vi "Actor Core.vi"(8 "error in":errorcluster, 11 "Create Test Channel View in":refnum<class "Create Test Channel View.lvclass">) -> (0 "error out":errorcluster, 3 "Actor out":refnum<class "Actor.lvclass">)   [LabVIEW 2013, in "Create Test Channel View.lvlib" / "Create Test Channel View.lvclass"]
doc: "(<B>Filename</B>: Actor Framework.lvlib:Actor.lvclass:Actor Core.vi)\n\nReceives messages to the actor, reacts to them, and initiates any error handling that may shut the actor down.\n\nDescendant classes may override this VI to append parallel tasks for the actor to complete while it handles messages. Overrides use the Call Parent Method node."
uses:
  Create Test Channel View.lvclass
  <vilib>/ActorFramework/Actor/Actor.lvclass
  <vilib>/ActorFramework/Actor/Actor.lvclass/Actor.ctl
  <vilib>/ActorFrameworkMVC/View Actor/View Actor.lvclass
  <vilib>/ActorFramework/Message Enqueuer/Message Enqueuer.lvclass/Message Enqueuer.ctl
  Create Test Channel View.lvclass/Create Test Channel View.ctl
  <vilib>/Utility/miscctls.llb/LVPositionTypeDef.ctl
  <vilib>/ActorFrameworkMVC/UI Controller Messages/Move Subpanel Msg/Move Subpanel Msg.lvclass/Move Subpanel Msg.ctl
  <vilib>/ActorFrameworkMVC/UI Controller Messages/Insert Subpanel Msg/Insert Subpanel Msg.lvclass/Insert Subpanel Msg.ctl
  Models/Create Test Channel Model Messages/Set Item Configurations Msg/Set Item Configurations Msg.lvclass/Set Item Configurations Msg.ctl
  <vilib>/ActorFramework/Message Enqueuer/Init from Existing Queue.vi
  <vilib>/ActorFramework/Message Enqueuer/Enqueue.vi
  <vilib>/ActorFramework/Message Priority Queue/Priority Enqueue.vi
  <vilib>/ActorFramework/Message Enqueuer/Message Enqueuer.lvclass
  <vilib>/ActorFrameworkMVC/UI Controller Messages/Move Subpanel Msg/Move Subpanel Msg.lvclass
  <vilib>/ActorFrameworkMVC/UI Controller Messages/Insert Subpanel Msg/Insert Subpanel Msg.lvclass
  Models/Create Test Channel Model Messages/Set Item Configurations Msg/Set Item Configurations Msg.lvclass
  Models/Create Test Channel Model Messages/Create Test Channel Msg/Create Test Channel Msg.lvclass
  Models/Test Channel Model Messages/Preview Test Channel Msg/Preview Test Channel Msg.lvclass
  Models/Test Channel Model Messages/Update Tiles Info Msg/Update Tiles Info Msg.lvclass
  Models/Test Channel Model Messages/Update Previous Button Visibility Msg/Update Previous Button Visibility Msg.lvclass
  Models/Test Channel Model Messages/Update Next Button Visibility Msg/Update Next Button Visibility Msg.lvclass
  Common/File IO/File IO.lvlib
  <vilib>/ActorFrameworkMVC/View Actor Messages/Get Model Enqueuer Msg/Get Model Enqueuer Msg.lvclass
  <vilib>/ActorFrameworkMVC/UI Controller Messages/Get Model Actor Enqueuer Msg/Get Model Actor Enqueuer Msg.lvclass
panel:
  in  "Cancel":bool
  in  "Save":bool
  out "Tab Control":enum32{"Basic Info"}(tab)
  in  "Channel Description":string caption="测试通道描述："
  in  "Channel Name":string caption="测试通道名称："
  in  "Channel ID":u16(ring) caption="测试通道ID：" items=["通道 1", "通道 2", "通道 3", "通道 4"]
  in  "Channel Sensor Name":u16(ring) caption="测试通道传感器：" items=["传感器 1", "传感器 2", "传感器 3", "传感器 4"]
  # "新建测试通道"
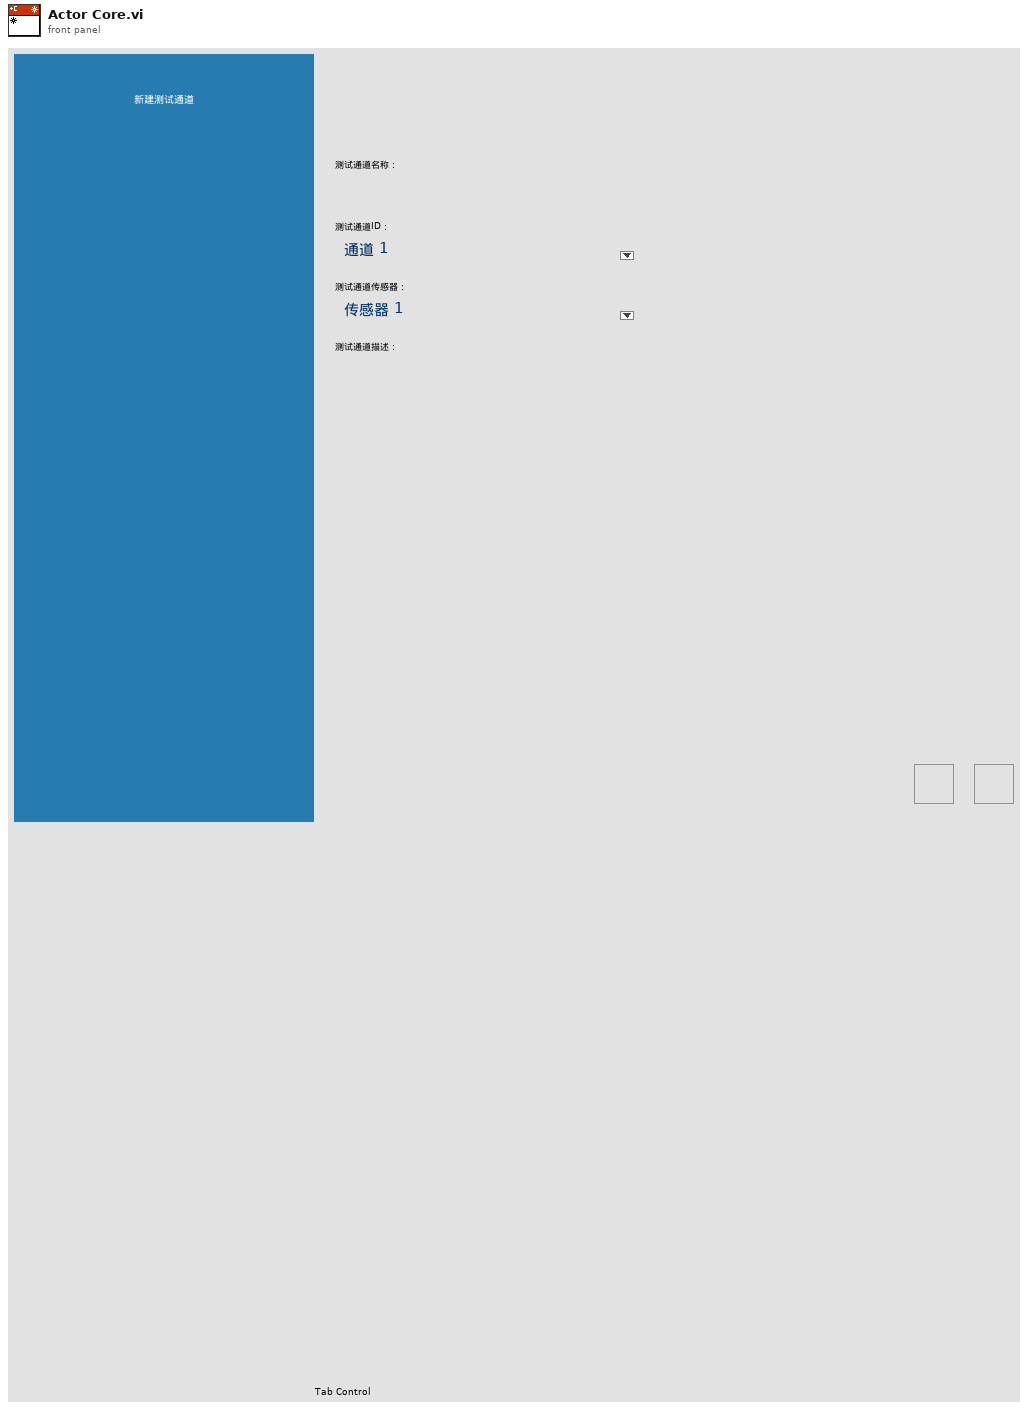
[diagram p1: front panel]
types:
  T1 = typedef "Create Test Channel View.lvlib/Create Test Channel View.lvclass/Events.ctl" = cluster{"Reinitialize All":refnum<user-event>, "Key Focus":refnum<user-event>, "Update Sensor Names":refnum<user-event>}
  T2 = typedef "LVPositionTypeDef.ctl" = cluster{"Left":i32, "Top":i32}
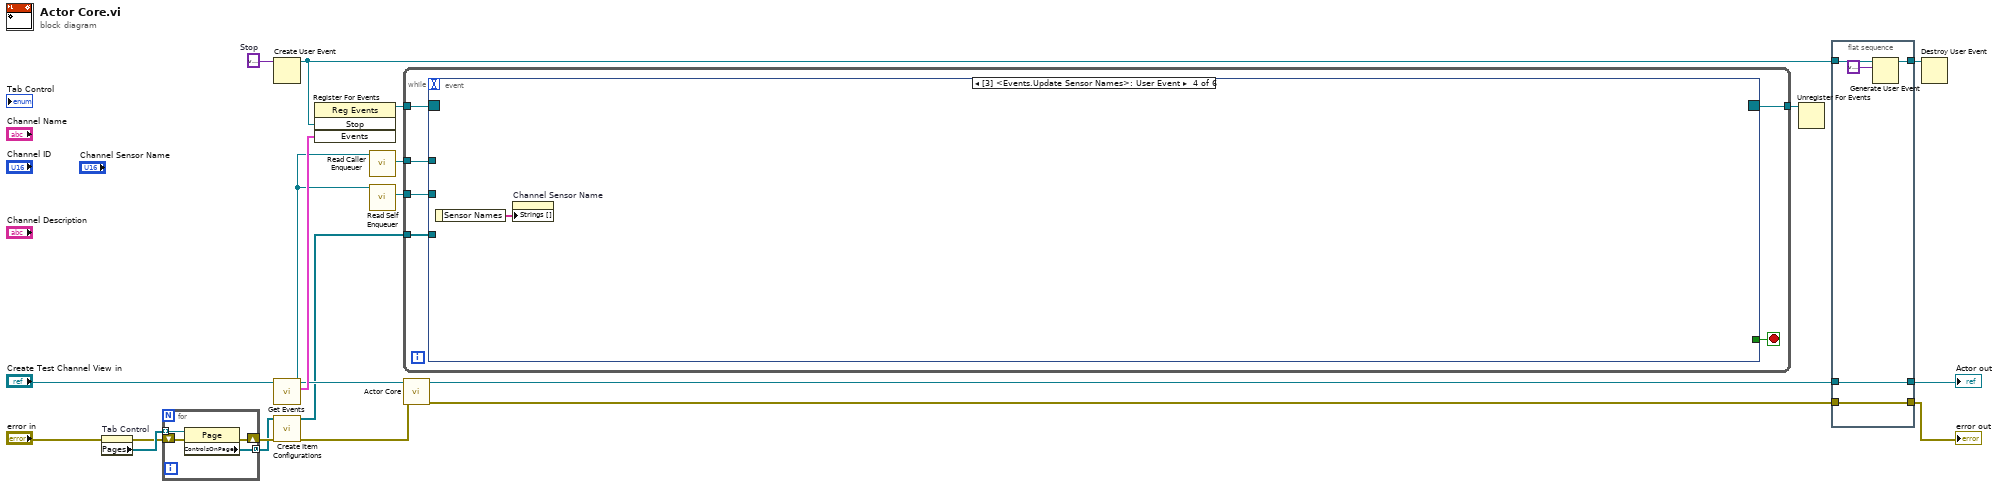
[diagram p0: block diagram]
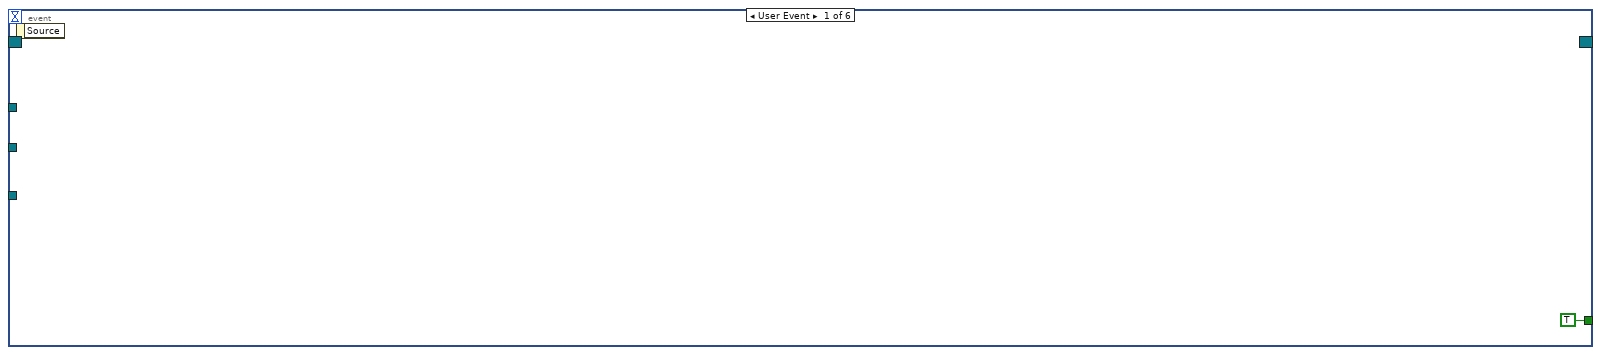
[diagram p2: hidden frame]
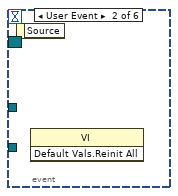
[diagram p3: hidden frame]
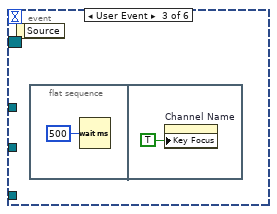
[diagram p4: hidden frame]
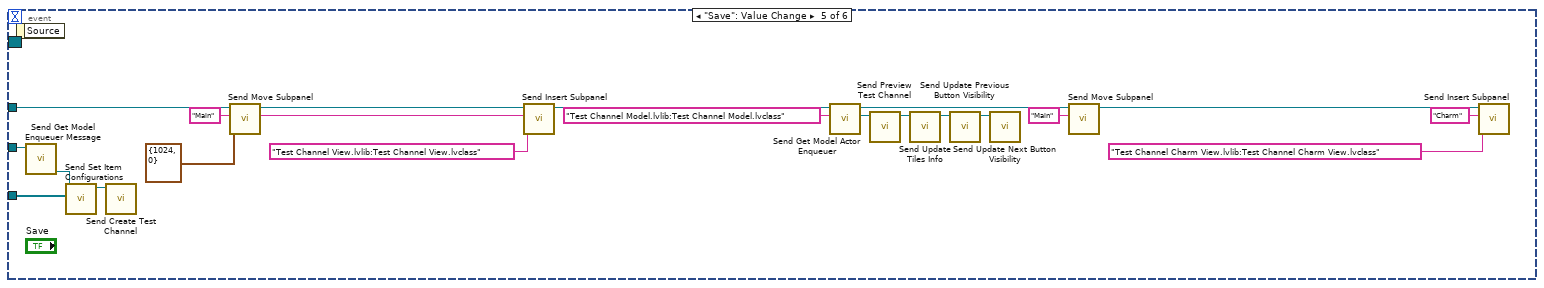
[diagram p5: hidden frame]
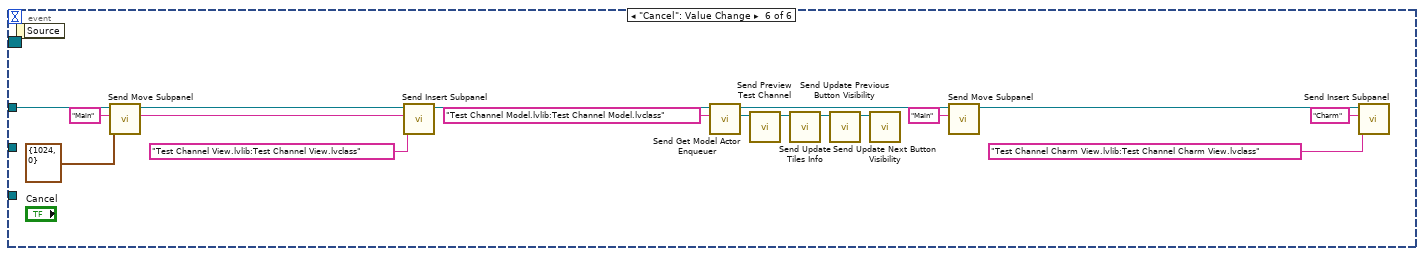
[diagram p6: hidden frame]
diagram:
  w21 = variant  # Stop
  n1 = property on="Tab Control" class="TabCtl (strict)"(error in="error in") -> (error out=w10:errorcluster, "Pages"=w11:refnum<vi>[])  [unwired: 1 in, 1 out]
  n2 = for {
    tunnel: w11 -> [w25] mode=indexing
    tunnel: [w24] -> w8 mode=concatenating
    shift-right: [w22] -> w9
    shift-left: w10 -> [w23]
    n3 = property class="Page"(reference=w25, error in=w23) -> (error out=w22:errorcluster, "ControlsOnPage"=w24:refnum<vi>[])  [unwired: 1 out]
  }
  n4 = Create User Event(user event datatype=w21) -> (user event=w14:refnum<user-event>)  [unwired: 1 in, 1 out]
  n5 = call "Get Events.vi"("Create Test Channel View in"="Create Test Channel View in") -> ("Events"=w13:T1, "Create Test Channel View out"=w4:refnum<class "Create Test Channel View.lvclass">)  [unwired: 9 in]
  n6 = call "Create Item Configurations.vi"("error in (no error)"=w9, "Controls References"=w8) -> ("error out"=w3:errorcluster, "Item Configurations"=w1:refnum<class "Item Configuration.lvclass">[])  [unwired: 8 in]
  n7 = register-events(w14, w13) -> (reference out=w15:refnum<event-registration>)  [unwired: 2 in, 1 out]
  n8 = call <vilib>:"Read Caller Enqueuer.vi"("Actor"=w4) -> ("Caller Enqueuer"=w6:refnum<class "Message Enqueuer.lvclass">)  [unwired: 10 in]
  n9 = call <vilib>:"Read Self Enqueuer.vi"("Actor"=w4) -> ("Self Enqueuer"=w5:refnum<class "Message Enqueuer.lvclass">)  [unwired: 10 in]
  n10 = while {
    tunnel: [w31] -> w12
    tunnel: w15 -> [w29]
    tunnel: w6 -> [w28]
    tunnel: w5 -> [w27]
    tunnel: w1 -> [w26]
    stop <- w30 stop-if-true
    n11 = event shown="[3] <Events.Update Sensor Names>: User Event" {
      selector: w29 -> [_ _ _ _ _ _]
      dyn-events: [_ _ _ _ _ _] -> w31
      timeout: _ -> [_ _ _ _ _ _]
      tunnel: [TRUE _ _ _ _ _] -> w30
      tunnel: w28 -> [_ _ _ _ w48 w68]
      tunnel: w27 -> [_ _ _ _ w53 _]
      tunnel: w26 -> [_ _ _ _ w52 _]
      event User Event {
        n12 = event-data() -> ()  [unwired: 1 in, 1 out]
      }
      event User Event {
        n13 = event-data() -> ()  [unwired: 1 in, 1 out]
        n14 = invoke class="VI" method="Default Vals.Reinit All"() -> ()  [unwired: 3 in, 3 out]
      }
      event User Event {
        n15 = event-data() -> ()  [unwired: 1 in, 1 out]
        n16 = flat-sequence {
          frame #0 {
            n17 = Wait (ms)(milliseconds to wait=u32 500) -> ()  [unwired: 1 out]
          }
          frame #1 {
            n18 = property on="Channel Name" class="Str"("Key Focus"=TRUE) -> ()  [unwired: 2 in, 2 out]
          }
        }
      }
      event User Event {
        n19 = event-data() -> ("Sensor Names"=w35:string[])  [unwired: 1 in]
        n20 = property on="Channel Sensor Name" class="Ring (strict)"("Strings []"=w35) -> ()  [unwired: 2 in, 2 out]
      }
      event "Save": Value Change {
        w38 = "Main" ("Subpanel Name")
        n21 = event-data() -> ()  [unwired: 1 in, 1 out]
        n22 = call <vilib>:"Send Get Model Enqueuer Message.vi"("Message Enqueuer in"=w53) -> ("Reply"=w55:refnum<class "Message Enqueuer.lvclass">)  [unwired: 7 in, 3 out]
        n23 = call "Send Set Item Configurations.vi"("Item Configurations"=w52, "Message Enqueuer"=w55) -> ("Message Enqueuer out"=w54:refnum<class "Message Enqueuer.lvclass">)  [unwired: 8 in, 1 out]
        n24 = call "Send Create Test Channel.vi"("Message Enqueuer"=w54) -> ()  [unwired: 9 in, 2 out]
        n25 = call <vilib>:"Send Move Subpanel.vi"("Position (0,0)"=T2 {"Left"=1024, "Top"=0}, "Subpanel Name"=w38, "Message Enqueuer"=w48) -> ("Message Enqueuer out"=w40:refnum<class "Message Enqueuer.lvclass">)  [unwired: 7 in, 1 out]
        n26 = call <vilib>:"Send Insert Subpanel.vi"("View Name"="Test Channel View.lvlib:Test Channel View.lvclass" ("Subpanel Name"), "Subpanel Name"=w38, "Message Enqueuer"=w40) -> ("Message Enqueuer out"=w45:refnum<class "Message Enqueuer.lvclass">)  [unwired: 7 in, 1 out]
        n27 = call <vilib>:"Send Get Model Actor Enqueuer.vi"("Model Name"="Test Channel Model.lvlib:Test Channel Model.lvclass", "Message Enqueuer in"=w45) -> ("Reply"=w41:refnum<class "Message Enqueuer.lvclass">, "Message Enqueuer out"=w39:refnum<class "Message Enqueuer.lvclass">)  [unwired: 6 in, 2 out]
        n28 = call "Send Preview Test Channel.vi"("Message Enqueuer"=w41) -> ("Message Enqueuer out"=w44:refnum<class "Message Enqueuer.lvclass">)  [unwired: 9 in, 1 out]
        n29 = call "Send Update Tiles Info.vi"("Message Enqueuer"=w44) -> ("Message Enqueuer out"=w43:refnum<class "Message Enqueuer.lvclass">)  [unwired: 9 in, 1 out]
        n30 = call "Send Update Previous Button Visibility.vi"("Message Enqueuer"=w43) -> ("Message Enqueuer out"=w42:refnum<class "Message Enqueuer.lvclass">)  [unwired: 9 in, 1 out]
        n31 = call "Send Update Next Button Visibility.vi"("Message Enqueuer"=w42) -> ()  [unwired: 9 in, 2 out]
        n32 = call <vilib>:"Send Move Subpanel.vi"("Subpanel Name"="Main", "Message Enqueuer"=w39) -> ("Message Enqueuer out"=w49:refnum<class "Message Enqueuer.lvclass">)  [unwired: 8 in, 1 out]
        n33 = call <vilib>:"Send Insert Subpanel.vi"("View Name"="Test Channel Charm View.lvlib:Test Channel Charm View.lvclass", "Subpanel Name"="Charm", "Message Enqueuer"=w49) -> ()  [unwired: 7 in, 2 out]
      }
      event "Cancel": Value Change {
        w58 = "Main" ("Subpanel Name")
        n34 = event-data() -> ()  [unwired: 1 in, 1 out]
        n35 = call <vilib>:"Send Move Subpanel.vi"("Position (0,0)"=T2 {"Left"=1024, "Top"=0}, "Subpanel Name"=w58, "Message Enqueuer"=w68) -> ("Message Enqueuer out"=w60:refnum<class "Message Enqueuer.lvclass">)  [unwired: 7 in, 1 out]
        n36 = call <vilib>:"Send Insert Subpanel.vi"("View Name"="Test Channel View.lvlib:Test Channel View.lvclass" ("Subpanel Name"), "Subpanel Name"=w58, "Message Enqueuer"=w60) -> ("Message Enqueuer out"=w65:refnum<class "Message Enqueuer.lvclass">)  [unwired: 7 in, 1 out]
        n37 = call <vilib>:"Send Get Model Actor Enqueuer.vi"("Model Name"="Test Channel Model.lvlib:Test Channel Model.lvclass", "Message Enqueuer in"=w65) -> ("Reply"=w61:refnum<class "Message Enqueuer.lvclass">, "Message Enqueuer out"=w59:refnum<class "Message Enqueuer.lvclass">)  [unwired: 6 in, 2 out]
        n38 = call "Send Preview Test Channel.vi"("Message Enqueuer"=w61) -> ("Message Enqueuer out"=w64:refnum<class "Message Enqueuer.lvclass">)  [unwired: 9 in, 1 out]
        n39 = call "Send Update Tiles Info.vi"("Message Enqueuer"=w64) -> ("Message Enqueuer out"=w63:refnum<class "Message Enqueuer.lvclass">)  [unwired: 9 in, 1 out]
        n40 = call "Send Update Previous Button Visibility.vi"("Message Enqueuer"=w63) -> ("Message Enqueuer out"=w62:refnum<class "Message Enqueuer.lvclass">)  [unwired: 9 in, 1 out]
        n41 = call "Send Update Next Button Visibility.vi"("Message Enqueuer"=w62) -> ()  [unwired: 9 in, 2 out]
        n42 = call <vilib>:"Send Move Subpanel.vi"("Subpanel Name"="Main", "Message Enqueuer"=w59) -> ("Message Enqueuer out"=w69:refnum<class "Message Enqueuer.lvclass">)  [unwired: 8 in, 1 out]
        n43 = call <vilib>:"Send Insert Subpanel.vi"("View Name"="Test Channel Charm View.lvlib:Test Channel Charm View.lvclass", "Subpanel Name"="Charm", "Message Enqueuer"=w69) -> ()  [unwired: 7 in, 2 out]
      }
    }
  }
  n44 = call-parent "Actor Core.vi"("error in"=w3, "View Actor in"=w4) -> ("error out"=w18:errorcluster, "Actor out"=w19:refnum<class "Actor.lvclass">)  [unwired: 8 in]
  n45 = Unregister For Events(event registration refnum=w12) -> ()  [unwired: 1 in, 1 out]
  n46 = flat-sequence "Generate a stop event when the actor core stopped." {
    tunnel: w14 -> [w76]
    tunnel: [w74] -> w20
    tunnel: w19 -> [w73]
    tunnel: w18 -> [w72]
    tunnel: [w73] -> w17
    tunnel: [w72] -> w16
    frame #0 {
      n47 = Generate User Event(user event=w76, event data cluster=variant ("event data")) -> (user event out=w74:refnum<user-event>)  [unwired: 2 in, 1 out]
    }
  }
  n48 = Destroy User Event(user event=w20) -> ()  [unwired: 1 in, 1 out]
  "error out" <- w16
  "Actor out" <- w17
